vi "Init.vi"(8 "error in (no error)":errorcluster, 10 "Node Reg":refnum<k20>, 11 "Node in":refnum<class "Node.lvclass">) -> (0 "error out":errorcluster, 3 "Node out":refnum<class "Node.lvclass">)   [LabVIEW 2025, in "Node.lvclass"]
uses:
  Node.lvclass
  Node.lvclass/Node.ctl
  Controls/Terminal.ctl
  <vilib>/xml/NI_XML.lvlib
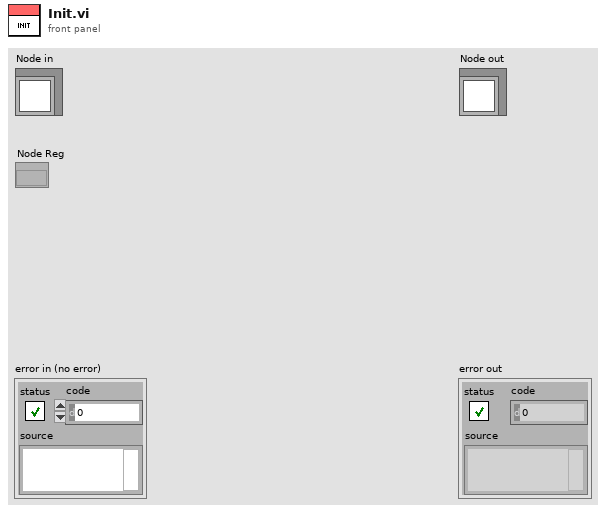
[diagram p1: front panel]
types:
  T1 = typedef "Terminal.ctl" = cluster{"id":string, "name":string, "terminal":refnum<vi>}
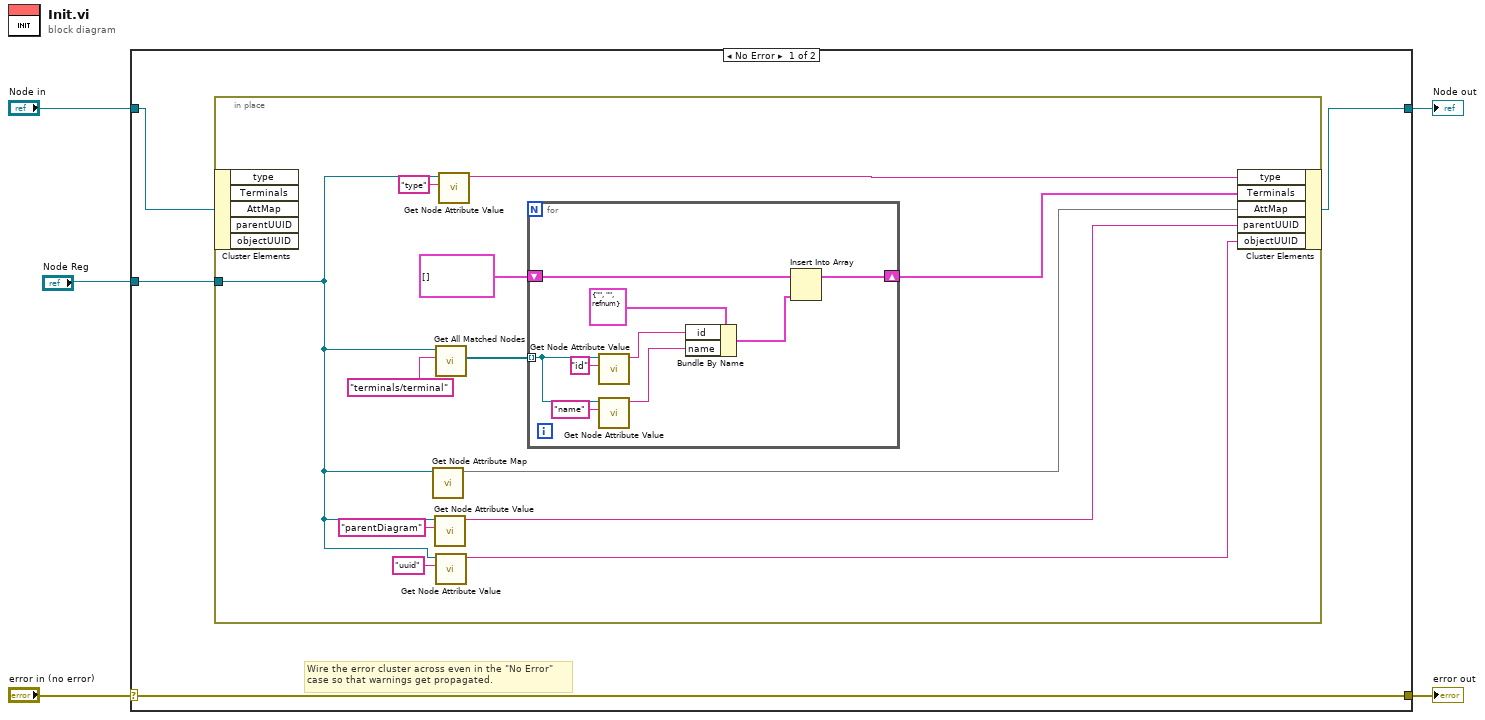
[diagram p0: block diagram]
diagram:
  n1 = case shown="No Error" "error in (no error)" {
    selector: "error in (no error)" -> [w9 w32]
    tunnel: [w9 w32] -> w4
    tunnel: [w6 w31] -> w2
    tunnel: "Node in" -> [w8 w31]
    tunnel: "Node Reg" -> [w7 _]
    frame No Error {
      # "Wire the error cluster across even in the \"No Error\"\ncase so that warnings get propagated."
      n2 = in-place {
        in-place-border: w7 -> [w11]
        n3 = in-place-cluster #1(w8) -> ()  [unwired: 5 out]
        n4 = call "Get Node Attribute Map.vi"("Refnum in"=w11) -> ("Map"=w20:map{string, string})  [unwired: 10 in]
        n5 = call "Get Node Attribute Value.vi"("Attribute Name"="parentDiagram", "Refnum in"=w11) -> ("Value"=w13:string)  [unwired: 9 in]
        n6 = call <vilib>:"Get All Matched Nodes.vi"("XPath expression"="terminals/terminal", "node in"=w11) -> ("node result array"=w17:refnum<k20>[])  [unwired: 7 in, 2 out]
        n7 = call "Get Node Attribute Value.vi"("Attribute Name"="uuid", "Refnum in"=w11) -> ("Value"=w10:string)  [unwired: 9 in]
        n8 = call "Get Node Attribute Value.vi"("Attribute Name"="type", "Refnum in"=w11) -> ("Value"=w19:string)  [unwired: 9 in]
        n9 = for {
          tunnel: w17 -> [w28] mode=indexing
          shift-right: [w29] -> w15
          shift-left: T1[] [] ("Terminals") -> [w30]
          n10 = call "Get Node Attribute Value.vi"("Attribute Name"="id", "Refnum in"=w28) -> ("Value"=w23:string)  [unwired: 9 in]
          n11 = call "Get Node Attribute Value.vi"("Attribute Name"="name", "Refnum in"=w28) -> ("Value"=w22:string)  [unwired: 9 in]
          n12 = Bundle By Name(cluster=T1 {"id"="", "name"="", "terminal"=refnum} ("Terminal"), "id"=w23, "name"=w22) -> (w24:T1)
          n13 = Insert Into Array(array=w30, new element=w24) -> (w29:T1[])  [unwired: 1 in]
        }
        n14 = in-place-cluster #1("type"=w19, "Terminals"=w15, "AttMap"=w20, "parentUUID"=w13, "objectUUID"=w10) -> (w6:refnum<class "Node.lvclass">)
      }
    }
    frame Error {
    }
  }
  "error out" <- w4
  "Node out" <- w2
